vi "Destructor.vi"(8 "error in":errorcluster, 11 "IntergerMeasure":refnum<class "IntegerMeasure.lvclass">) -> (0 "error out":errorcluster)   [LabVIEW 2021, in "ProligentXMLGenerator.lvlib" / "IntegerMeasure.lvclass"]
uses:
  IntegerMeasure.lvclass
  IntegerMeasure.lvclass/IntegerMeasure.ctl
  Measure/Measure.lvclass
  MeasureLimit/MeasureLimit.lvclass
  IntegerMeasureLimit/IntegerMeasureLimit.lvclass
  C:/Projects/proligent-xml-generator-labview/src/ProligentXMLGenerator/Measure/Measure/Measure.lvclass
  C:/Projects/proligent-xml-generator-labview/src/ProligentXMLGenerator/Measure/IntegerMeasure/IntegerMeasure.lvclass
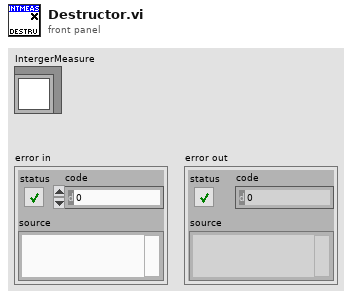
[diagram p1: front panel]
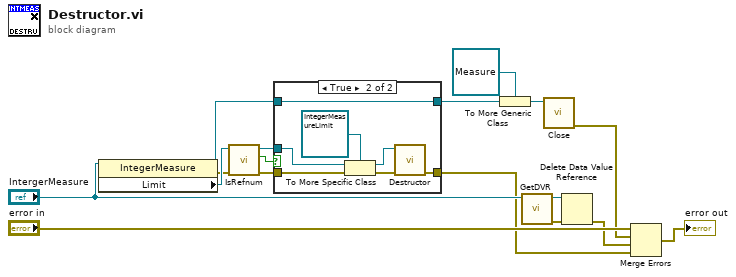
[diagram p0: block diagram]
diagram:
  n1 = property class="IntegerMeasure"(reference="IntergerMeasure") -> (reference out=w4:refnum<class "IntegerMeasure.lvclass">, error out=w6:errorcluster, "Limit"=w7:refnum<class "MeasureLimit.lvclass">)  [unwired: 1 in]
  n2 = call "IsRefnum.vi"("error in"=w6, "MeasureLimit in"=w7) -> ("error out"=w10:errorcluster, "IsRefnum"=w8:bool, "MeasureLimit out"=w9:refnum<class "MeasureLimit.lvclass">)  [unwired: 7 in]
  n3 = case shown="True" w8 {
    tunnel: w10 -> [w19 w25]
    tunnel: w9 -> [_ w24]
    tunnel: [w19 w22] -> w2
    tunnel: [w18 w26] -> w5
    tunnel: w4 -> [w18 w26]
    frame False {
    }
    frame True {
      n4 = To More Specific Class(target class=refnum<class "IntegerMeasureLimit.lvclass"> refnum ("ProligentResultProcessor:IntegerMeasureLimit"), reference=w24, error in=w25) -> (specific class reference=w21:refnum<class "IntegerMeasureLimit.lvclass">, error out=w23:errorcluster)
      n5 = call "Destructor.vi"("error in"=w23, "IntegerMeasureLimit"=w21) -> ("error out"=w22:errorcluster)  [unwired: 9 in]
    }
  }
  n6 = To More Generic Class(target class=refnum<class "Measure.lvclass"> refnum ("ProligentResultProcessor:Measure"), reference=w5) -> (generic class reference=w3:refnum<class "Measure.lvclass">)
  n7 = call "GetDVR.vi"("IntergerMeasure"="IntergerMeasure") -> ("error out"=w14:errorcluster, "DVRReference"=w15:refnum<data-value>)  [unwired: 9 in]
  n8 = call "Close.vi"("Measure"=w3) -> ("error out"=w1:errorcluster)  [unwired: 10 in]
  n9 = Delete Data Value Reference(data value reference=w15, error in=w14) -> (error out=w13:errorcluster)  [unwired: 1 out]
  n10 = Merge Errors("error in", w1, w13, w2) -> (→"error out":errorcluster)
